vi "Get Next Direction.vi"(8 "error in (no error)":errorcluster, 11 "Application in":refnum<class "Game.lvclass">) -> (0 "error out":errorcluster, 1 "Direction":T1, 3 "Application out":refnum<class "Game.lvclass">)   [LabVIEW 2021, in "Game.lvclass"]
doc: "Wait for next movement event to move the snake."
uses:
  Game.lvclass
  GameEl_class/private/Enum Direction.ctl
  Game.lvclass/Game.ctl
  GameEl_class/GameEl.lvclass
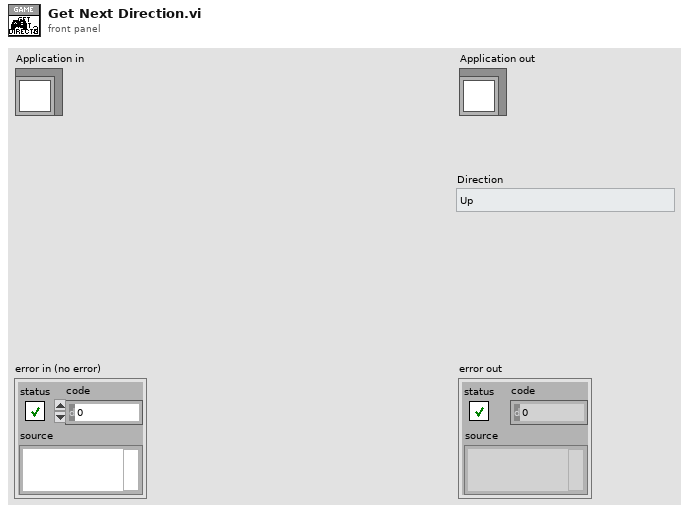
[diagram p1: front panel]
types:
  T1 = typedef "GameEl.lvclass/Enum Direction.ctl" = enum16{"Up", "Down", "Forward", "Backward"}
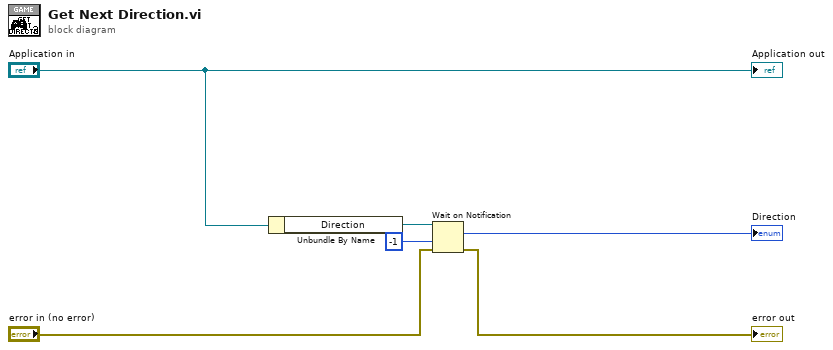
[diagram p0: block diagram]
diagram:
  n1 = Unbundle By Name("Application in") -> ("Direction"=w2:refnum<notifier>)
  n2 = Wait on Notification(notifier=w2, timeout in ms (-1)=-1, error in (no error)="error in (no error)") -> (notification=→"Direction":T1, error out=→"error out":errorcluster)  [unwired: 1 in, 2 out]
  "Application out" <- "Application in"
